vi "q3 y1 y2 plot.vi"() -> ()   [LabVIEW 2018]
panel:
  out "X":dbl
  out "Y2":dbl
  out "Y1":dbl
  out "XY Graph":cluster{dbl, dbl, dbl}[](graph)
  in  "h":dbl
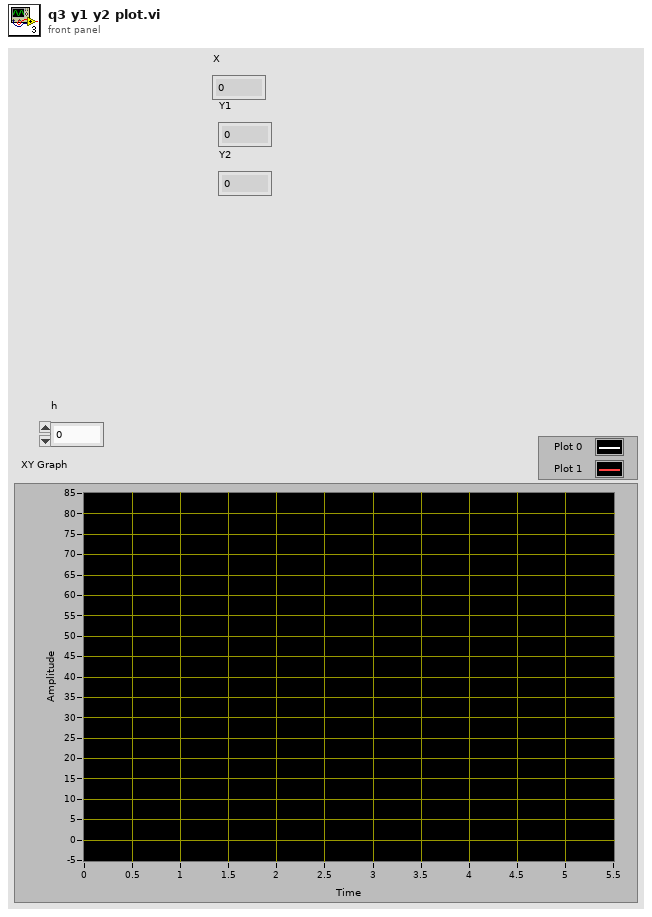
[diagram p1: front panel]
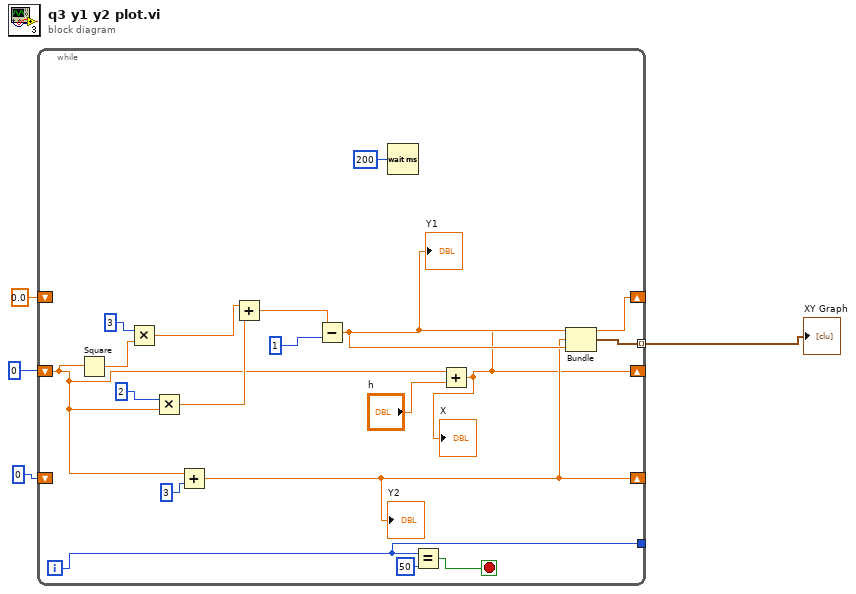
[diagram p0: block diagram]
diagram:
  n1 = while {
    shift-right: [w6] -> _
    shift-left: 0 -> [w12]
    shift-right: [w9] -> _
    shift-left: 0.0 -> [_]
    shift-right: [w8] -> _
    shift-left: 0 -> [_]
    tunnel: [w10] -> _
    tunnel: [w7] -> w1 mode=indexing
    i -> [w10]
    stop <- w22 stop-if-true
    n2 = Square(x=w12) -> (x^2=w19:dbl)
    n3 = Multiply(x=3, y=w19) -> (x*y=w17:dbl)
    n4 = Multiply(x=2, y=w12) -> (x*y=w16:dbl)
    n5 = Add(x=w12, y=3) -> (x+y=w8:dbl)
    "Y2" <- w8
    n6 = Add(x=w17, y=w16) -> (x+y=w15:dbl)
    n7 = Subtract(x=w15, y=1) -> (x-y=w9:dbl)
    "Y1" <- w9
    n8 = Wait (ms)(milliseconds to wait=200) -> ()  [unwired: 1 out]
    n9 = Equal?(x=w10, y=50) -> (x = y?=w22:bool)
    n10 = Add(x=w12, y="h") -> (x+y=w6:dbl)
    "X" <- w6
    n11 = Bundle(w6, w8, w9) -> (w7:cluster{dbl, dbl, dbl})  [unwired: 1 in]
  }
  "XY Graph" <- w1
